vi "Finish.vi"   [LabVIEW 2016]
doc: "This VI is called just before exiting. It is expected to close I/O refnum, save collected data, etc."
uses:
  <vilib>/Rock Robotics/WPI/Utilities/WPI_GetSetVariantRefNum.vi
types:
  T1 = typedef "WPI_RobotDriveDevRef.ctl" = cluster{"DevStatus":errorcluster, "Motors[]":T2[], "Square Inputs":bool, "Max Output":dbl}
  T2 = typedef "WPI_MotorControlDeviceRef.ctl" = cluster{"DeviceStatus":errorcluster, "Type":T3, "PWM":cluster{"PWM Channel":T4, "DeadBand":T5}, "CAN":cluster{"Device Number":u8, "SetOutput VI Ref":variant, "GetOutput VI Ref":variant, "Enable VI Ref":variant, "Disable VI Ref":variant, "Data":variant}, "Invert":bool}
  T3 = typedef "WPI_MotorControlType.ctl" = enum16{"PWM", "CAN"}
  T4 = typedef "FPGA_DIOPWMChannel.ctl" = enum8{"PWM 0", "PWM 1", "PWM 2", "PWM 3", "PWM 4", "PWM 5", "PWM 6", "PWM 7", "PWM 8", "PWM 9", "PWM MXP 0", "PWM MXP 1", "PWM MXP 2", "PWM MXP 3", "PWM MXP 4", "PWM MXP 5", "PWM MXP 6", "PWM MXP 7", "PWM MXP 8", "PWM MXP 9", "Invalid"}
  T5 = typedef "WPI_PWMDeadband.ctl" = cluster{"Name":string, "maxPositivePwm":i32, "minPositivePwm":i32, "centerPwm":i32, "maxNegativePwm":i32, "minNegativePwm":i32, "angularRange":u16}
  T6 = typedef "WPI_EncoderDevRef.ctl" = cluster{"DevStatus":errorcluster, "EncoderIndex":T7, "CounterIndex":T8, "DistancePerCount":dbl, "Decoding Type":T9}
  T7 = typedef "FPGA_EncoderIdx.ctl" = enum8{"Enc 0", "Enc 1", "Enc 2", "Enc 3", "Enc 4", "Enc 5", "Enc 6", "Enc 7", "Invalid"}
  T8 = typedef "FPGA_CounterCtrSystemIndex.ctl" = enum8{"Ctr 0", "Ctr 1", "Ctr 2", "Ctr 3", "Ctr 4", "Ctr 5", "Ctr 6", "Ctr 7", "Invalid"}
  T9 = typedef "WPI_EncoderType.ctl" = enum16{"1x", "2x", "4x"}
  T10 = typedef "WPI_JoystickDevRef.ctl" = cluster{"Device":T11}
  T11 = typedef "WPI_JoystickDeviceEnum.ctl" = enum16{"USB 0", "USB 1", "USB 2", "USB 3", "USB 4", "USB 5"}
  T12 = typedef "WPI_DigitalInputDevRef.ctl" = cluster{"DevStatus":errorcluster, "DIO Channel":T13}
  T13 = typedef "FPGA_DIOChannel.ctl" = enum8{"DIO 0", "DIO 1", "DIO 2", "DIO 3", "DIO 4", "DIO 5", "DIO 6", "DIO 7", "DIO 8", "DIO 9", "DIO MXP 0", "DIO MXP 1", "DIO MXP 2", "DIO MXP 3", "DIO MXP 4", "DIO MXP 5", "DIO MXP 6", "DIO MXP 7", "DIO MXP 8", "DIO MXP 9", "DIO MXP 10", "DIO MXP 11", "DIO MXP 12", "DIO MXP 13", "DIO MXP 14", "DIO MXP 15", "SPI Port CS1", "SPI Port CS2", "SPI Port CS3", "SPI Port MISO", "SPI Port MOSI", "Invalid"}
  T14 = typedef "WPI_SolenoidDevRef.ctl" = cluster{"DevStatus":errorcluster, "Pneumatics Control Module":u8, "Forward Solenoid Channel":T15, "Reverse Solenoid Channel":T15}
  T15 = typedef "WPI_SolenoidChannel.ctl" = enum8{"Solenoid 0", "Solenoid 1", "Solenoid 2", "Solenoid 3", "Solenoid 4", "Solenoid 5", "Solenoid 6", "Solenoid 7", "Invalid"}
  T16 = typedef "WPI_CameraDevRef.ctl" = cluster{"Camera Address":string, "CameraStatus":errorcluster}
  T17 = typedef "WPI_SwitchDevRef.ctl" = cluster{"DevStatus":errorcluster, "DIO Channel":T13, "CntIndex":T8, "Normally Closed":bool}
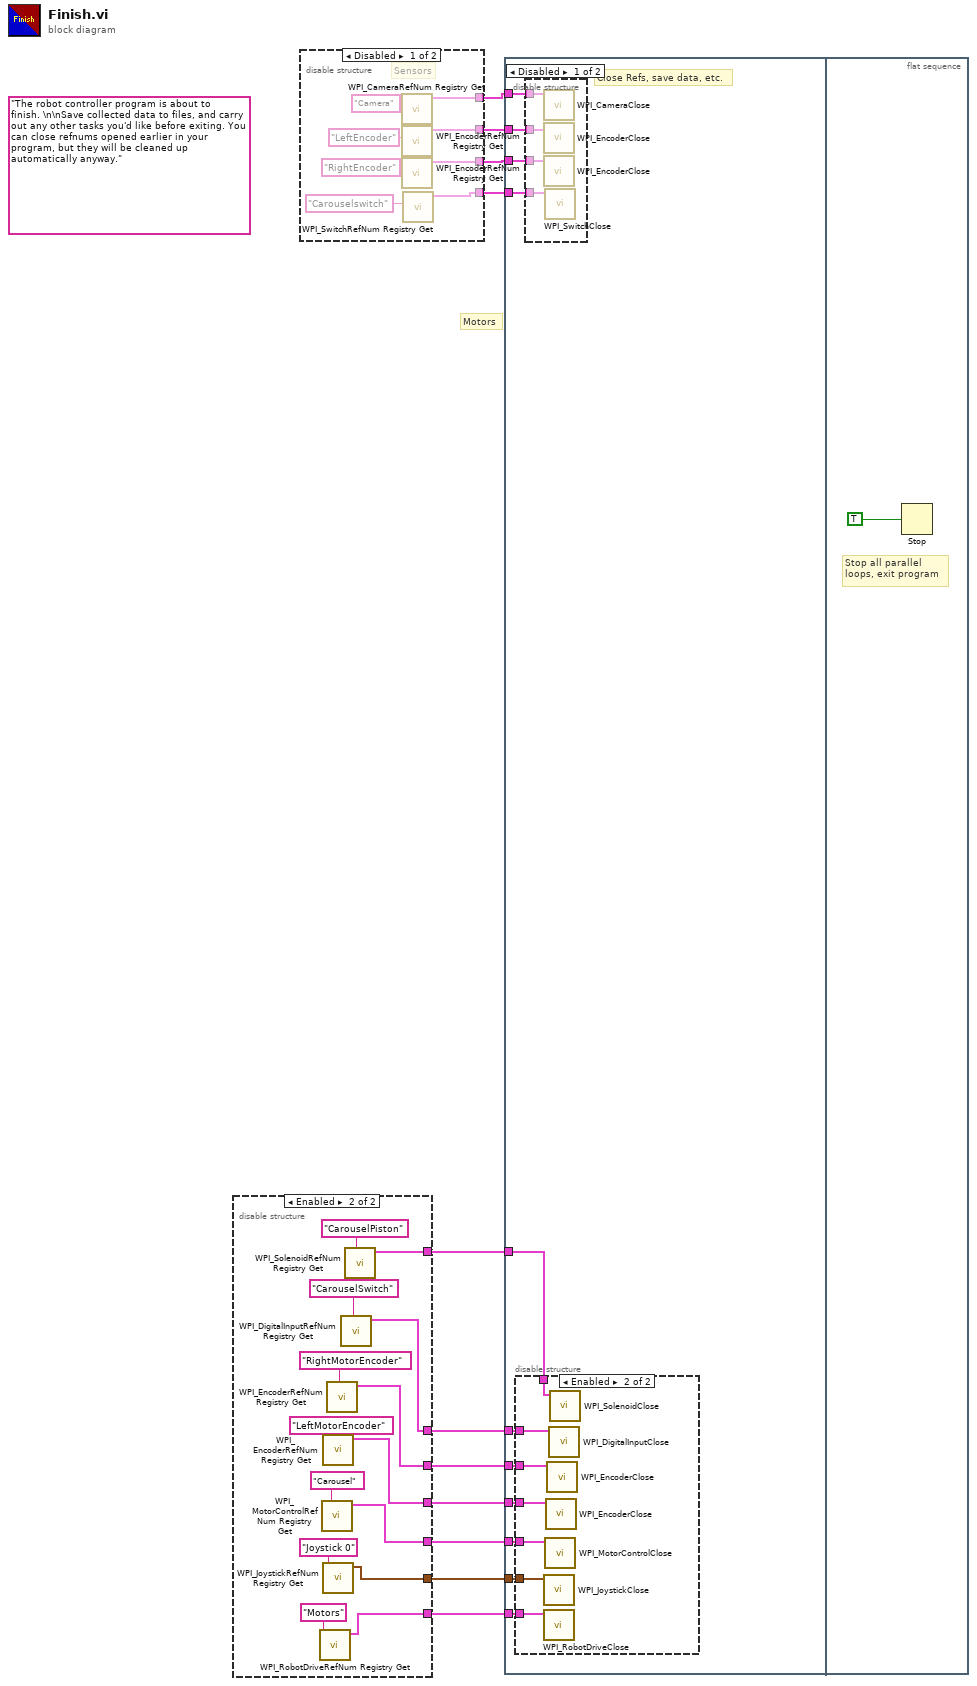
[diagram p0: block diagram]
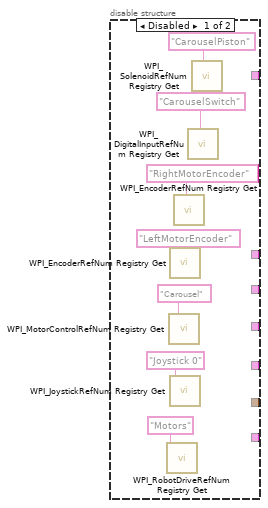
[diagram p3: hidden frame]
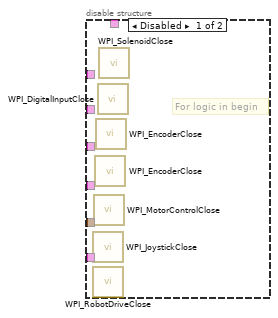
[diagram p5: hidden frame]
diagram:
  (unwired) "The robot controller program is about to finish. \n\nSave collected data to files, and carry out any other tasks you'd like before exiting. You can close refnums opened earlier in your program, but they will be cleaned up automatically anyway."
  # "Motors"
  n1 = disable-structure shown="Enabled" {
    disable-tunnel: [_ w25] -> w7
    disable-tunnel: [_ w24] -> w6
    disable-tunnel: [_ w23] -> w5
    disable-tunnel: [_ w22] -> w4
    disable-tunnel: [_ w21] -> w3
    disable-tunnel: [_ w20] -> w2
    disable-tunnel: [_ w19] -> w1
    frame Disabled {
      n2 = call <vilib>:"WPI_RobotDriveRefNum Registry Get.vi"("refnum name"="Motors") -> ()  [unwired: 1 in, 10 out]
      n3 = call <vilib>:"WPI_MotorControlRefNum Registry Get.vi"("refnum name"="Carousel") -> ()  [unwired: 9 in, 2 out]
      n4 = call <vilib>:"WPI_EncoderRefNum Registry Get.vi"("refnum name"="LeftMotorEncoder") -> ()  [unwired: 9 in, 2 out]
      n5 = call <vilib>:"WPI_JoystickRefNum Registry Get.vi"("refnum name"="Joystick 0") -> ()  [unwired: 1 in, 10 out]
      n6 = call <vilib>:"WPI_EncoderRefNum Registry Get.vi"("refnum name"="RightMotorEncoder") -> ()  [unwired: 9 in, 2 out]
      n7 = call <vilib>:"WPI_DigitalInputRefNum Registry Get.vi"("refnum name"="CarouselSwitch") -> ()  [unwired: 9 in, 2 out]
      n8 = call <vilib>:"WPI_SolenoidRefNum Registry Get.vi"("refnum name"="CarouselPiston") -> ()  [unwired: 9 in, 2 out]
    }
    frame Enabled {
      n9 = call <vilib>:"WPI_RobotDriveRefNum Registry Get.vi"("refnum name"="Motors") -> ("RobotDriveDevRef"=w19:T1)  [unwired: 1 in, 9 out]
      n10 = call <vilib>:"WPI_MotorControlRefNum Registry Get.vi"("refnum name"="Carousel") -> ("MotorControlDevRef"=w21:T2)  [unwired: 9 in, 1 out]
      n11 = call <vilib>:"WPI_EncoderRefNum Registry Get.vi"("refnum name"="LeftMotorEncoder") -> ("EncoderDevRef"=w22:T6)  [unwired: 9 in, 1 out]
      n12 = call <vilib>:"WPI_JoystickRefNum Registry Get.vi"("refnum name"="Joystick 0") -> ("JoystickDevRef"=w20:T10)  [unwired: 1 in, 9 out]
      n13 = call <vilib>:"WPI_EncoderRefNum Registry Get.vi"("refnum name"="RightMotorEncoder") -> ("EncoderDevRef"=w23:T6)  [unwired: 9 in, 1 out]
      n14 = call <vilib>:"WPI_DigitalInputRefNum Registry Get.vi"("refnum name"="CarouselSwitch") -> ("DigitalInputDevRef"=w24:T12)  [unwired: 9 in, 1 out]
      n15 = call <vilib>:"WPI_SolenoidRefNum Registry Get.vi"("refnum name"="CarouselPiston") -> ("SolenoidDevRef"=w25:T14)  [unwired: 9 in, 1 out]
    }
  }
  n16 = disable-structure shown="Disabled" {
    disable-tunnel: [w40 _] -> w11
    disable-tunnel: [w38 _] -> w10
    disable-tunnel: [w35 _] -> w9
    disable-tunnel: [w34 _] -> w8
    frame Disabled {
      # "Sensors"
      n17 = call <vilib>:"WPI_CameraRefNum Registry Get.vi"("refnum name"="Camera") -> ("CameraDevRef"=w40:T16)  [unwired: 9 in, 1 out]
      n18 = call <vilib>:"WPI_EncoderRefNum Registry Get.vi"("refnum name"="LeftEncoder") -> ("EncoderDevRef"=w38:T6)  [unwired: 9 in, 1 out]
      n19 = call <vilib>:"WPI_EncoderRefNum Registry Get.vi"("refnum name"="RightEncoder") -> ("EncoderDevRef"=w35:T6)  [unwired: 9 in, 1 out]
      n20 = call <vilib>:"WPI_SwitchRefNum Registry Get.vi"("refnum name"="Carouselswitch") -> ("SwitchDevRef"=w34:T17)  [unwired: 9 in, 1 out]
    }
    frame Enabled {
    }
  }
  n21 = flat-sequence {
    tunnel: w11 -> [w51]
    tunnel: w10 -> [w50]
    tunnel: w9 -> [w49]
    tunnel: w8 -> [w48]
    tunnel: w7 -> [w47]
    tunnel: w6 -> [w46]
    tunnel: w5 -> [w45]
    tunnel: w4 -> [w44]
    tunnel: w3 -> [w43]
    tunnel: w2 -> [w42]
    tunnel: w1 -> [w41]
    frame #0 {
      # "Close Refs, save data, etc."
      n22 = disable-structure shown="Enabled" {
        disable-tunnel: w47 -> [_ w62]
        disable-tunnel: w46 -> [_ w61]
        disable-tunnel: w45 -> [_ w60]
        disable-tunnel: w44 -> [_ w59]
        disable-tunnel: w43 -> [_ w58]
        disable-tunnel: w42 -> [_ w57]
        disable-tunnel: w41 -> [_ w56]
        frame Disabled {
          # "For logic in begin"
          n23 = call <vilib>:"WPI_JoystickClose.vi"() -> ()  [unwired: 1 in, 11 out]
          n24 = call <vilib>:"WPI_RobotDriveClose.vi"() -> ()  [unwired: 2 in, 10 out]
          n25 = call <vilib>:"WPI_MotorControlClose.vi"() -> ()  [unwired: 11 in, 1 out]
          n26 = call <vilib>:"WPI_EncoderClose.vi"() -> ()  [unwired: 11 in, 1 out]
          n27 = call <vilib>:"WPI_EncoderClose.vi"() -> ()  [unwired: 11 in, 1 out]
          n28 = call <vilib>:"WPI_DigitalInputClose.vi"() -> ()  [unwired: 11 in, 1 out]
          n29 = call <vilib>:"WPI_SolenoidClose.vi"() -> ()  [unwired: 11 in, 1 out]
        }
        frame Enabled {
          n30 = call <vilib>:"WPI_JoystickClose.vi"("JoystickDevRef"=w57) -> ()  [unwired: 11 out]
          n31 = call <vilib>:"WPI_RobotDriveClose.vi"("RobotDriveDevRef"=w56) -> ()  [unwired: 1 in, 10 out]
          n32 = call <vilib>:"WPI_MotorControlClose.vi"("MotorControlDevRef"=w58) -> ()  [unwired: 10 in, 1 out]
          n33 = call <vilib>:"WPI_EncoderClose.vi"("EncoderDevRef"=w59) -> ()  [unwired: 10 in, 1 out]
          n34 = call <vilib>:"WPI_EncoderClose.vi"("EncoderDevRef"=w60) -> ()  [unwired: 10 in, 1 out]
          n35 = call <vilib>:"WPI_DigitalInputClose.vi"("DigitalInputDevRef"=w61) -> ()  [unwired: 10 in, 1 out]
          n36 = call <vilib>:"WPI_SolenoidClose.vi"("SolenoidDevRef"=w62) -> ()  [unwired: 10 in, 1 out]
        }
      }
      n37 = disable-structure shown="Disabled" {
        disable-tunnel: w51 -> [w55 _]
        disable-tunnel: w50 -> [w54 _]
        disable-tunnel: w49 -> [w53 _]
        disable-tunnel: w48 -> [w52 _]
        frame Disabled {
          n38 = call <vilib>:"WPI_CameraClose.vi"("CameraDevRef"=w55) -> ()  [unwired: 10 in, 1 out]
          n39 = call <vilib>:"WPI_EncoderClose.vi"("EncoderDevRef"=w54) -> ()  [unwired: 10 in, 1 out]
          n40 = call <vilib>:"WPI_EncoderClose.vi"("EncoderDevRef"=w53) -> ()  [unwired: 10 in, 1 out]
          n41 = call <vilib>:"WPI_SwitchClose.vi"("SwitchDevRef"=w52) -> ()  [unwired: 10 in, 1 out]
        }
        frame Enabled {
        }
      }
    }
    frame #1 {
      # "Stop all parallel\nloops, exit program"
      n42 = Stop(stop? (T)=TRUE ("Quit")) -> ()
    }
  }
